vi "sound.vi"(8 "error in (no error)":errorcluster caption="错误输入（无错误）", 11 "dog 输入":refnum<class "dog.lvclass">) -> (0 "error out":errorcluster caption="错误输出", 3 "dog 输出":refnum<class "dog.lvclass">)   [LabVIEW 2018, in "dog.lvclass"]
uses:
  dog.lvclass
  animal.lvclass
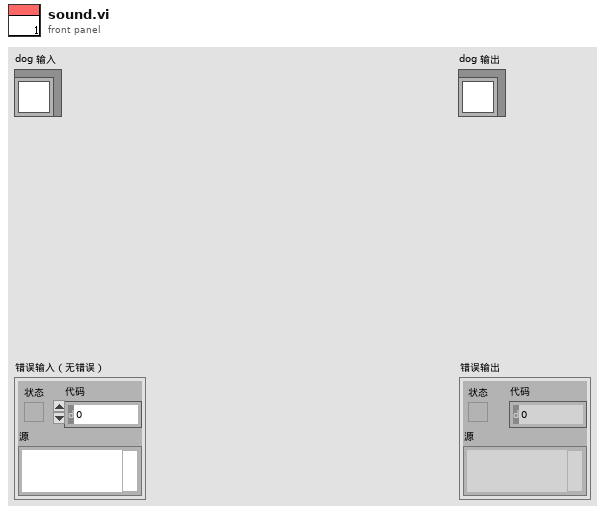
[diagram p1: front panel]
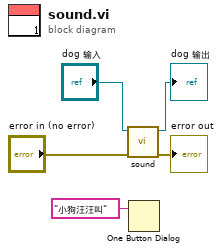
[diagram p0: block diagram]
diagram:
  n1 = call-parent "sound.vi"("error in (no error)"="error in (no error)", "animal 输入"="dog 输入") -> ("error out"=→"error out":errorcluster, "animal 输出"=→"dog 输出":refnum<class "dog.lvclass">)  [unwired: 8 in]
  n2 = One Button Dialog(message="小狗汪汪叫" ("消息")) -> ()  [unwired: 1 in, 1 out]
